vi "GetCurrentSquare.vi"(8 "error in (no error)":errorcluster, 11 "object in":refnum<class "Piece.lvclass">) -> (0 "error out":errorcluster, 1 "Current Square":cluster{"Column":string, "Row":i32}, 2 "currentSquare":map{string, i32}(c390), 3 "object out":refnum<class "Piece.lvclass">, 5 "Row":i32, 7 "Column (Numeric)":u8)   [LabVIEW 2020, in "Piece.lvclass"]
uses:
  Piece.lvclass
  Piece.lvclass/Piece.ctl
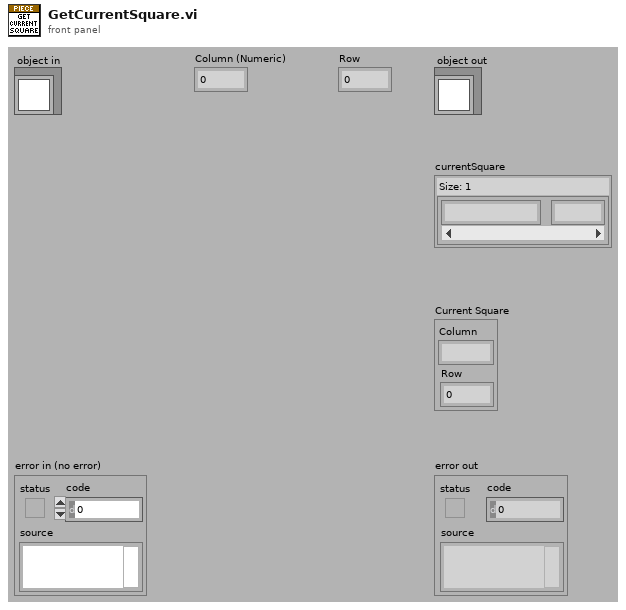
[diagram p1: front panel]
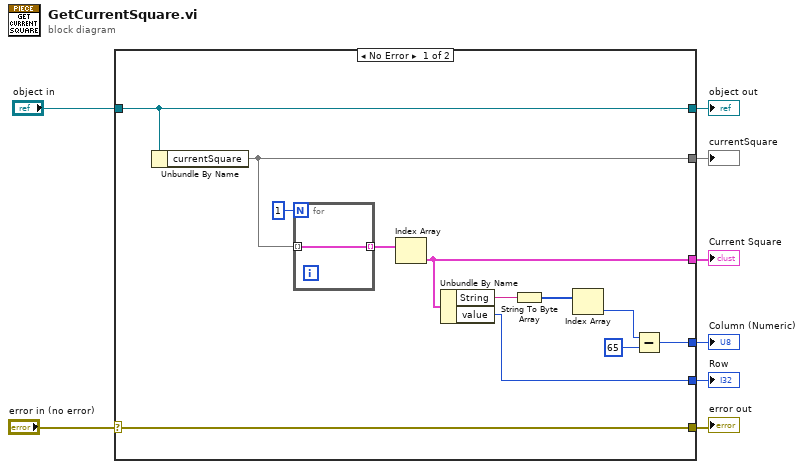
[diagram p0: block diagram]
diagram:
  n1 = case shown="No Error" "error in (no error)" {
    selector: "error in (no error)" -> [w20 w23]
    tunnel: [w20 w23] -> w7
    tunnel: [w19 w22] -> w5
    tunnel: "object in" -> [w19 w22]
    tunnel: [w16 _] -> w4
    tunnel: [w15 _] -> w3
    tunnel: [w10 _] -> w2
    tunnel: [w9 _] -> w1
    frame No Error {
      n2 = Unbundle By Name(w19) -> ("currentSquare"=w16:map{string, i32})
      n3 = for {
        N: 1 -> [_]
        tunnel: [w21] -> w17 mode=indexing
        tunnel: w16 -> [w21] mode=indexing
      }
      n4 = Index Array(array=w17) -> (element=w15:cluster{"String":string, "value":i32})  [unwired: 1 in]
      n5 = Unbundle By Name(w15) -> ("String"=w14:string, "value"=w9:i32)
      n6 = String To Byte Array(string=w14) -> (unsigned byte array=w13:u8[])
      n7 = Index Array(array=w13) -> (element=w12:u8)  [unwired: 1 in]
      n8 = Subtract(x=w12, y=u8 65) -> (x-y=w10:u8)
    }
    frame Error {
    }
  }
  "error out" <- w7
  "object out" <- w5
  "currentSquare" <- w4
  "Current Square" <- w3
  "Column (Numeric)" <- w2
  "Row" <- w1
